vi "PathSettingDialog.vi"(0 "Path in":T1={"TS file"=path "C:/Users/lpnhe/Desktop/Labview/damic/DAMIC-LTC/DamicLTC-seul-Essai.txt", "Log file"=path "C:/DAMIC/DAMIC-LTC/Data/log.txt", "Log Directory"=path "C:/DAMIC/DAMIC-LTC/Data", "Output aspic file folder"=path "C:/Users/lpnhe/Desktop/Labview/damic/DAMIC-LTC/Data", "TSfile folder"=path "C:/Users/lpnhe/Desktop/Labview/damic/DAMIC_TIMESLICE"}, 5 "error in (no error)":errorcluster) -> (14 "Path out":T1={"TS file"=path "C:/Users/lpnhe/Desktop/Labview/damic/DAMIC-LTC/DamicLTC-seul-Essai.txt", "Log file"=path "C:/DAMIC/DAMIC-LTC/Data/log.txt", "Log Directory"=path "C:/DAMIC/DAMIC-LTC/Data", "Output aspic file folder"=path "C:/Users/lpnhe/Desktop/Labview/damic/DAMIC-LTC/Data", "TSfile folder"=path "C:/Users/lpnhe/Desktop/Labview/damic/DAMIC_TIMESLICE"}, 17 "UI Refresh Needed ?":bool, 19 "error out":errorcluster)   [LabVIEW 2014]
uses:
  path.ctl
panel:
  out "TSfile folder":path
  out "Output aspic file folder":path
  out "Log Directory":path
  out "Log file":path
  out "TS file":path
  in  "TSfile folder":path=path "C:/Users/lpnhe/Desktop/Labview/damic/DAMIC_TIMESLICE"
  in  "Output aspic file folder":path=path "C:/Users/lpnhe/Desktop/Labview/damic/DAMIC-LTC/Data"
  in  "Log Directory":path=path "C:/DAMIC/DAMIC-LTC/Data"
  in  "Log file":path=path "C:/DAMIC/DAMIC-LTC/Data/log.txt"
  in  "TS file":path=path "C:/Users/lpnhe/Desktop/Labview/damic/DAMIC-LTC/DamicLTC-seul-Essai.txt"
  in  "Cancel Button":bool
  in  "OK Button":bool
  # "Path settings"
  # "TO set path"
  # "Current path"
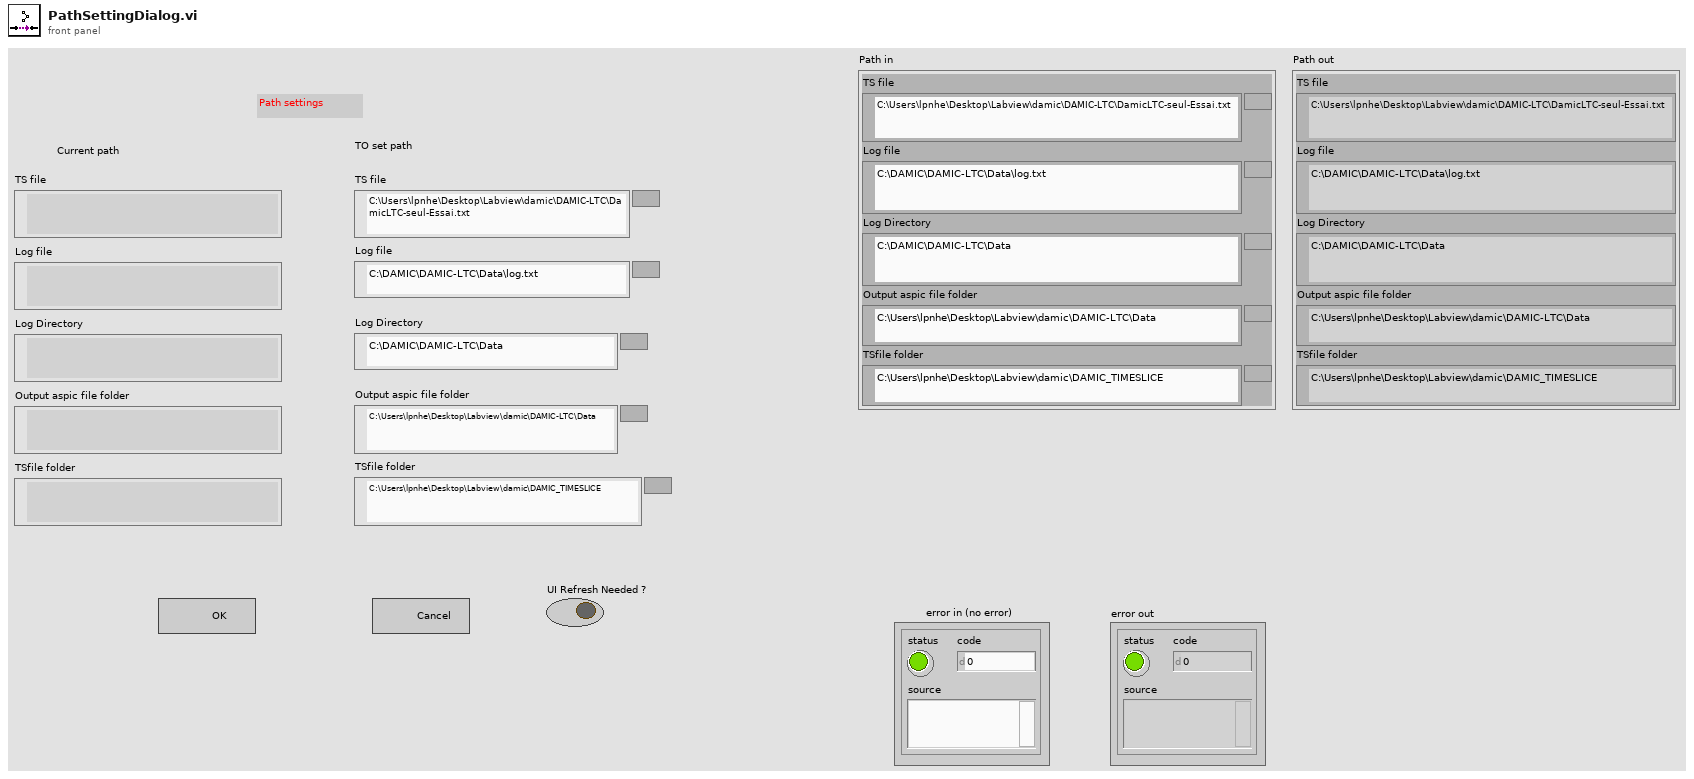
[diagram p1: front panel]
types:
  T1 = typedef "path.ctl" = cluster{"TS file":path, "Log file":path, "Log Directory":path, "Output aspic file folder":path, "TSfile folder":path}
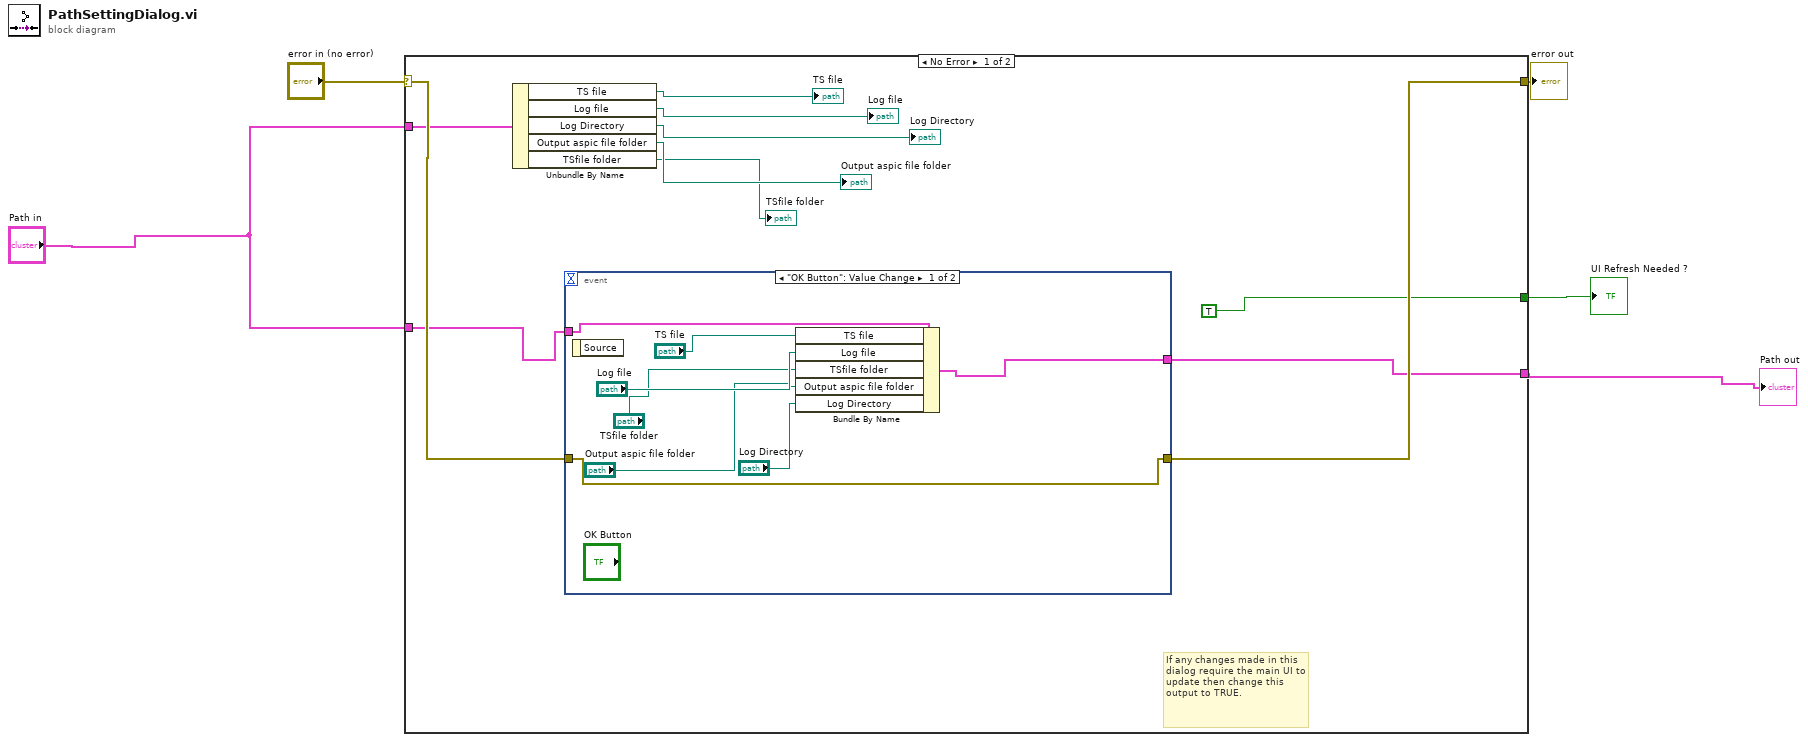
[diagram p0: block diagram]
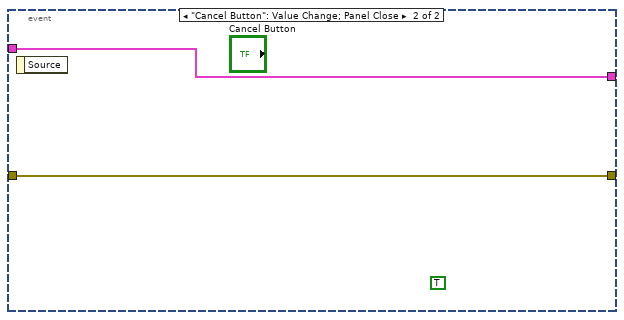
[diagram p2: hidden frame]
diagram:
  n1 = case shown="No Error" "error in (no error)" {
    selector: "error in (no error)" -> [w16 w27]
    tunnel: [w15 w27] -> w5
    tunnel: [w14 _] -> w2
    tunnel: "Path in" -> [w13 _]
    tunnel: "Path in" -> [w12 _]
    tunnel: [TRUE _] -> w1
    frame No Error {
      # "If any changes made in this dialog require the main UI to update then change this output to TRUE."
      n2 = Unbundle By Name(w13) -> ("TS file"=→"TS file":path, "Log file"=→"Log file":path, "Log Directory"=→"Log Directory":path, "Output aspic file folder"=→"Output aspic file folder":path, "TSfile folder"=→"TSfile folder":path)
      n3 = event shown="[0] \"OK Button\": Value Change" {
        selector: _ -> [_ _]
        dyn-events: _ -> [_ _]
        timeout: _ -> [_ _]
        tunnel: [w18 w26] -> w14
        tunnel: w12 -> [w24 w26]
        tunnel: w16 -> [w17 w25]
        tunnel: [w17 w25] -> w15
        event "OK Button": Value Change {
          n4 = event-data() -> ()  [unwired: 1 in, 1 out]
          n5 = Bundle By Name(cluster=w24, "TS file"="TS file", "Log file"="Log file", "TSfile folder"="TSfile folder", "Output aspic file folder"="Output aspic file folder", "Log Directory"="Log Directory") -> (w18:T1)
        }
        event "Cancel Button": Value Change; Panel Close {
          (unwired) TRUE
          n6 = event-data() -> ()  [unwired: 1 in, 1 out]
        }
      }
    }
    frame Error {
    }
  }
  "UI Refresh Needed ?" <- w1
  "error out" <- w5
  "Path out" <- w2
